vi "example test.vi"() -> ()   [LabVIEW 2013, in "CVT tests.lvlib"]
uses:
  CVT tests.lvlib
  execution/CVT runtime.lvclass
  configuration/CVT configuration.lvclass
  <vilib>/NI/Tag Bus/tag/Data Type.ctl
  <vilib>/NI/Tag Bus Module Framework/channel/channel classification.ctl
  <vilib>/NI/Tag Bus/dictionary/data dictionary.lvclass/data dictionary.ctl
  <vilib>/NI/Tag Bus/dictionary/lookup polymorphs/locate double.vi
  <vilib>/NI/Tag Bus/table/data polymorphs/write one/write Double.vi
  <vilib>/NI/Tag Bus/table/data polymorphs/read one/read Double.vi
  <vilib>/NI/Tag Bus/dictionary/search/find data index.vi
  <vilib>/NI/Tag Bus/dictionary/search/search string list.vi
  <vilib>/NI/Tag Bus/dictionary/tag not found.vi
  <vilib>/NI/Tag Bus Module Framework/channel/TBM channel.lvclass
  <vilib>/NI/Tag Bus/tag/tag descriptor.lvclass
  <vilib>/NI/Tag Bus/dictionary/data dictionary.lvclass
  <vilib>/NI/Tag Bus/table/data table.lvlib
panel:
  in  "ch count":i32=100
  in  "for loop":i32=10000
  out "out usec/call":dbl
  out "in usec/call":dbl
  out "final error":errorcluster
  out "output error":errorcluster
  out "input error":errorcluster
  out "output lookup error":errorcluster
  out "no data written":bool
  out "input lookup error":errorcluster
  out "init error":errorcluster
  out "correct execution settings":bool
  out "serialization problem":errorcluster
  out "invalid configuration":errorcluster
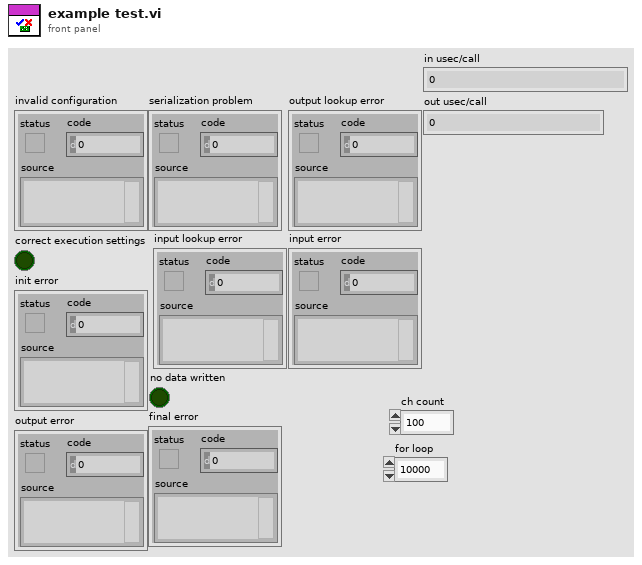
[diagram p1: front panel]
types:
  T1 = typedef "TBM channel.lvclass/channel classification.ctl" = enum16{"input data", "output data", "processing parameter", "processing result"}
  T2 = typedef "tag bus.lvlib/tag descriptor.lvclass/Data Type.ctl" = enum16{"Double", "Single", "I64", "I32", "I16", "I8", "U64", "U32", "U16", "U8", "Boolean", "String", "Array of Double", "Array of Single", "Array of I64", "Array of I32", "Array of I16", "Array of I8", "Array of U64", "Array of U32", "Array of U16", "Array of U8", "Array of Boolean", "Array of String"}
  T3 = typedef "TBM channel.lvclass/data tables.ctl" = cluster{"input data":T4, "processing parameter":T4, "processing result":T4, "output data":T4}
  T4 = typedef "tag bus.lvlib/dictionary table pair.ctl" = cluster{"data dictionary":refnum<class "data dictionary.lvclass">, "data table":T5}
  T5 = typedef "tag bus.lvlib/data table.lvlib/data table.ctl" = cluster{"Double":dbl[], "Single":sgl[], "I64":i64[], "I32":i32[], "I16":i16[], "I8":i8[], "U64":u64[], "U32":u32[], "U16":u16[], "U8":u8[], "Boolean":bool[], "String":string[], "Array of Double":cluster{"DBL Array":dbl[]}[], "Array of Single":cluster{"SGL Array":sgl[]}[], "Array of I64":cluster{"I64 Array":i64[]}[], "Array of I32":cluster{"I32 Array":i32[]}[], "Array of I16":cluster{"I16 Array":i16[]}[], "Array of I8":cluster{"I8 Array":i8[]}[], "Array of U64":cluster{"U64 Array":u64[]}[], "Array of U32":cluster{"U32 Array":u32[]}[], "Array of U16":cluster{"U16 Array":u16[]}[], "Array of U8":cluster{"U8 Array":u8[]}[], "Array of Boolean":cluster{"Boolean Array":bool[]}[], "Array of String":cluster{"String Array":string[]}[]}
  T6 = typedef "TBM module execution interface.lvclass/execution settings.ctl" = cluster{"reads inputs":bool, "processes data":bool, "writes outputs":bool}
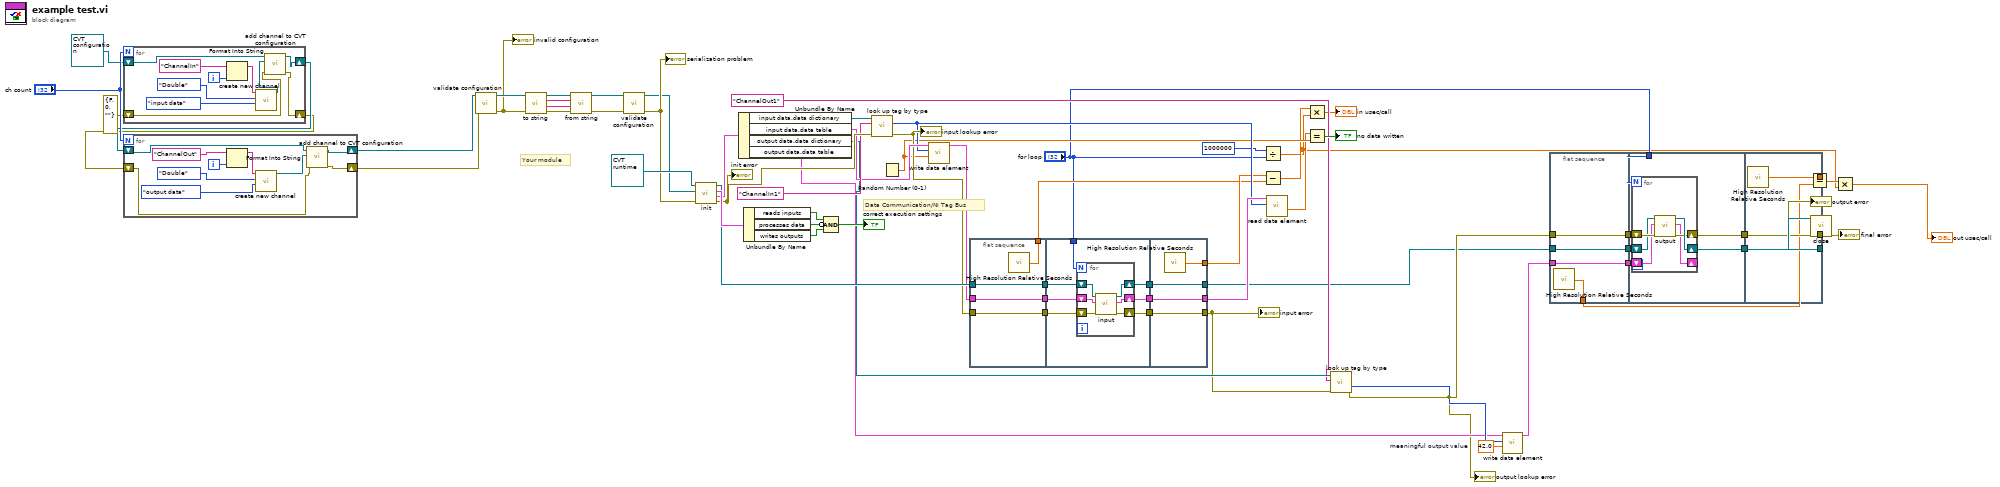
[diagram p0: block diagram]
diagram:
  w36 = 42.0  # meaningful output value
  # "Data Communication/NI Tag Bus"
  # "Your module"
  n1 = for {
    N: "ch count" -> [_]
    shift-right: [w74] -> w5
    shift-left: refnum<class "CVT configuration.lvclass"> refnum ("tag bus configurable plugin module configuration") -> [w73]
    shift-right: [w75] -> w2
    shift-left: errorcluster {"status"=FALSE, "code"=0, "source"=""} ("error out") -> [w71]
    i -> [w78]
    n2 = Format Into String(initial string="ChannelIn" ("channel name"), w78) -> (resulting string=w77:string)  [unwired: 2 in, 1 out]
    n3 = call <vilib>:"create new channel.vi"("channel classification"=channel_classification."input data", "data type"=Data_Type."Double", "channel name"=w77) -> ("channel"=w72:refnum<class "TBM channel.lvclass">)  [unwired: 8 in]
    n4 = call "add channel to CVT configuration.vi"("error in"=w71, "channel"=w72, "CVT configuration in"=w73) -> ("error out"=w75:errorcluster, "CVT configuration out"=w74:refnum<class "CVT configuration.lvclass">)  [unwired: 7 in]
  }
  n5 = for {
    N: "ch count" -> [_]
    shift-right: [w82] -> w4
    shift-left: w5 -> [w85]
    shift-right: [w83] -> w3
    shift-left: w2 -> [w84]
    i -> [w88]
    n6 = Format Into String(initial string="ChannelOut" ("channel name"), w88) -> (resulting string=w87:string)  [unwired: 2 in, 1 out]
    n7 = call <vilib>:"create new channel.vi"("channel classification"=channel_classification."output data", "data type"=Data_Type."Double", "channel name"=w87) -> ("channel"=w81:refnum<class "TBM channel.lvclass">)  [unwired: 8 in]
    n8 = call "add channel to CVT configuration.vi"("error in"=w84, "channel"=w81, "CVT configuration in"=w85) -> ("error out"=w83:errorcluster, "CVT configuration out"=w82:refnum<class "CVT configuration.lvclass">)  [unwired: 7 in]
  }
  n9 = call-dynamic "validate configuration.vi"("error in"=w3, "CVT configuration in"=w4) -> ("error out"=w69:errorcluster, "CVT configuration out"=w70:refnum<class "CVT configuration.lvclass">)  [unwired: 8 in]
  "invalid configuration" <- w69
  n10 = call-dynamic "to string.vi"("error in"=w69, "CVT configuration in"=w70) -> ("error out"=w65:errorcluster, "data"=w66:string, "version"=w67:string, "CVT configuration out"=w68:refnum<class "CVT configuration.lvclass">)  [unwired: 6 in]
  n11 = call-dynamic "from string.vi"("error in"=w65, "data"=w66, "version"=w67, "CVT configuration in"=w68) -> ("error out"=w63:errorcluster, "CVT configuration out"=w64:refnum<class "CVT configuration.lvclass">)  [unwired: 6 in]
  n12 = call-dynamic "validate configuration.vi"("error in"=w63, "CVT configuration in"=w64) -> ("error out"=w61:errorcluster, "CVT configuration out"=w60:refnum<class "CVT configuration.lvclass">)  [unwired: 8 in]
  "serialization problem" <- w61
  n13 = call-dynamic "init.vi"("error in"=w61, "TBM module configuration in"=w60, "CVT runtime in"=refnum<class "CVT runtime.lvclass"> refnum ("tag bus configurable plugin module")) -> ("error out"=w52:errorcluster, "data allocations"=w54:T3, "execution settings"=w59:T6, "CVT runtime out"=w49:refnum<class "CVT runtime.lvclass">)  [unwired: 5 in]
  "init error" <- w52
  n14 = Unbundle By Name(w54) -> ("input data.data dictionary"=w53:refnum<class "data dictionary.lvclass">, "input data.data table"=w50:T5, "output data.data dictionary"=w41:refnum<class "data dictionary.lvclass">, "output data.data table"=w38:T5)
  n15 = Unbundle By Name(w59) -> ("reads inputs"=w56:bool, "processes data"=w58:bool, "writes outputs"=w57:bool)
  n16 = Compound Arithmetic op=AND(w56, invert w58, w57) -> (→"correct execution settings":bool)
  n17 = call-poly <vilib>:"look up tag by type.vi"("error in"=w52, "name"="ChannelIn1" ("channel name"), "data dictionary in"=w53) -> ("error out"=w48:errorcluster, "index"=w45:i32)  [unwired: 6 in, 1 out]
  "input lookup error" <- w48
  n18 = Random Number (0-1)() -> (number: 0 to 1=w44:dbl)
  n19 = call-poly <vilib>:"write data element.vi"("value"=w44, "index"=w45, "data table in"=w50) -> ("data table out"=w47:T5)  [unwired: 8 in]
  n20 = flat-sequence {
    tunnel: w47 -> [w92]
    tunnel: w48 -> [w93]
    tunnel: w49 -> [w94]
    tunnel: [w94] -> w26
    tunnel: [w93] -> w25
    tunnel: [w92] -> w24
    tunnel: [w91] -> w22
    tunnel: [w98] -> w29
    tunnel: [w97] -> w28
    tunnel: [w96] -> w27
    tunnel: w26 -> [w101]
    tunnel: w25 -> [w100]
    tunnel: w24 -> [w99]
    tunnel: "for loop" -> [w95]
    tunnel: [w109] -> w34
    tunnel: [w110] -> w37
    tunnel: [w111] -> w46
    tunnel: w29 -> [w111]
    tunnel: w28 -> [w110]
    tunnel: w27 -> [w109]
    tunnel: [w108] -> w23
    frame #0 {
      n21 = call <vilib>:"High Resolution Relative Seconds.vi"() -> ("relative seconds"=w91:dbl)
    }
    frame #1 {
      n22 = for {
        N: w95 -> [_]
        shift-right: [w102] -> w96
        shift-left: w101 -> [w107]
        shift-right: [w104] -> w98
        shift-left: w99 -> [w105]
        shift-right: [w103] -> w97
        shift-left: w100 -> [w106]
        n23 = call-dynamic "input.vi"("error in"=w106, "data table in"=w105, "CVT runtime in"=w107) -> ("error out"=w103:errorcluster, "data table out"=w104:T5, "CVT runtime out"=w102:refnum<class "CVT runtime.lvclass">)  [unwired: 6 in]
      }
    }
    frame #2 {
      n24 = call <vilib>:"High Resolution Relative Seconds.vi"() -> ("relative seconds"=w108:dbl)
    }
  }
  n25 = Divide(x=1000000, y="for loop") -> (x/y=w9:dbl)
  n26 = Subtract(x=w23, y=w22) -> (x-y=w12:dbl)
  n27 = call-poly <vilib>:"read data element.vi"("index"=w45, "data table in"=w46) -> ("value"=w43:dbl)  [unwired: 8 in, 1 out]
  n28 = Multiply(x=w12, y=w9) -> (x*y=→"in usec/call":dbl)
  n29 = Equal?(x=w43, y=w44) -> (x = y?=→"no data written":bool)
  n30 = call-poly <vilib>:"look up tag by type.vi"("error in"=w37, "name"="ChannelOut1" ("channel name"), "data dictionary in"=w41) -> ("error out"=w35:errorcluster, "index"=w39:i32)  [unwired: 6 in, 1 out]
  "output lookup error" <- w35
  n31 = call-poly <vilib>:"write data element.vi"("value"=w36, "index"=w39, "data table in"=w38) -> ("data table out"=w33:T5)  [unwired: 8 in]
  n32 = flat-sequence {
    tunnel: w33 -> [w113]
    tunnel: w34 -> [w114]
    tunnel: w35 -> [w115]
    tunnel: [w115] -> w19
    tunnel: [w114] -> w18
    tunnel: [w113] -> w17
    tunnel: [w112] -> w15
    tunnel: [w118] -> w21
    tunnel: [w117] -> w20
    tunnel: w19 -> [w121]
    tunnel: w18 -> [w120]
    tunnel: w17 -> [w119]
    tunnel: "for loop" -> [w116]
    tunnel: [w129] -> w31
    tunnel: [w130] -> w32
    tunnel: w21 -> [w130]
    tunnel: w20 -> [w129]
    tunnel: [w128] -> w16
    frame #0 {
      n33 = call <vilib>:"High Resolution Relative Seconds.vi"() -> ("relative seconds"=w112:dbl)
    }
    frame #1 {
      n34 = for {
        N: w116 -> [_]
        shift-right: [w124] -> w118
        shift-left: w120 -> [w126]
        shift-right: [w123] -> w117
        shift-left: w121 -> [w127]
        shift-right: [w122] -> _
        shift-left: w119 -> [w125]
        n35 = call-dynamic "output.vi"("error in"=w127, "data table in"=w125, "CVT runtime in"=w126) -> ("error out"=w123:errorcluster, "data table out"=w122:T5, "CVT runtime out"=w124:refnum<class "CVT runtime.lvclass">)  [unwired: 6 in]
      }
    }
    frame #2 {
      n36 = call <vilib>:"High Resolution Relative Seconds.vi"() -> ("relative seconds"=w128:dbl)
    }
  }
  n37 = Subtract(x=w16, y=w15) -> (x-y=w10:dbl)
  n38 = call-dynamic "close.vi"("error in"=w31, "CVT runtime in"=w32) -> ("error out"=→"final error":errorcluster)  [unwired: 9 in]
  n39 = Multiply(x=w10, y=w9) -> (x*y=→"out usec/call":dbl)
  "input error" <- w37
  "output error" <- w31
